vi "blink led(SubVI).vi"(10 "Boolean in":bool, 11 "Numeric in":dbl) -> (3 "Boolean out":bool)   [LabVIEW 2017]
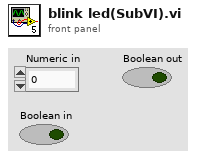
[diagram p1: front panel]
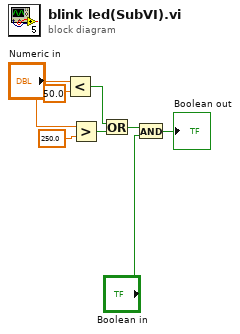
[diagram p0: block diagram]
diagram:
  n1 = Less?(x="Numeric in", y=50.0) -> (x < y?=w5:bool)
  n2 = Greater?(x="Numeric in", y=250.0) -> (0:w4:bool)
  n3 = Or(x=w5, y=w4) -> (x .or. y?=w7:bool)
  n4 = And(x=w7, y="Boolean in") -> (x .and. y?=→"Boolean out":bool)
